vi "Boolean to Checkbox Checked Attribute.vi"(0 "Boolean":bool) -> (2 "Checked Attribute":string)   [LabVIEW 2011]
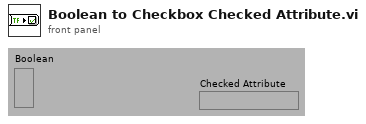
[diagram p1: front panel]
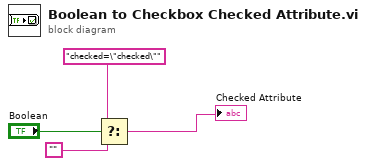
[diagram p0: block diagram]
diagram:
  n1 = Select(t="checked=\"checked\"", s="Boolean", f="") -> (s? t:f=→"Checked Attribute":string)
